vi "GeoFonu_v1.3.vi"() -> ()   [LabVIEW 2014]
uses:
  <vilib>/Instr/_visa.llb/VISA Set IO Buffer Mask.ctl
  <vilib>/Instr/_visa.llb/VISA Flush IO Buffer Mask.ctl
  <vilib>/Instr/_visa.llb/VISA Configure Serial Port (Instr).vi
panel:
  out "Sensor3":i32[](graph)=[342, 333, 338, 337, 336, 340, 338, 334, 337, 337, 333, 337, 339, 337, 337, 337, 317, 337, 334, 335, 338, 338, 316, 333, 339, 337, 338, 337, 338, 337, 337, 338, 335, 334, 338, 334, 337, 337, 338, 337, 337, 339, 335, 338, 337, 338, 337, 336, 334, 332, 338, 335, 337, 335, 334, 337, 337, 335, 338, 338, 335, 336, 338, 337, 337, 336, 337, 339, 337, 336, 338, 337, 337, 335, 334, 335, 337, 338, 329, 338, 337, 338, 339, 339, 335, 338, 337, 334, 351, 337, 328, 346, 336, 337, 336, 339, 336, 338, 335, 333, 337, 360, 338, 333, 338, 334, 339, 336, 336, 337, 336, 313, 339, 337, 337, 337, 304, 338, 338, 338, 336, 340, 336, 336, 338, 335, 338, 335, 338, 333, 329, 336, 342, 336, 335, 335, 338, 336, 336, 338, 334, 336, 336, 313, 337, 337, 334, 329, 338, 336, 329, 341, 336, 335, 336, 338, 332, 334, 337, 336, 336, 337, 334, 337, 336, 333, 336, 336, 338, 336, 337, 338, 342, 338, 344, 338, 343, 338, 338, 325, 336, 337, 337, 335, 338, 339, 337, 339, 336, 336, 336, 336, 332, 334, 338, 338, 339, 359, 339, 333, 337, 339, 333, 338, 337, 338, 336, 342, 338, 336, 336, 337, 334, 337, 337, 341, 335, 334, 338, 335, 341, 333, 336, 336, 330, 335, 336, 336, 331, 340, 336, 337, 334, 336, 336, 334, 341, 334, 336, 339, 338, 336, 336, 336, 335, 335, 336, 336, 337, 334, 336, 335, 339, 336, 334, 334, 338, 336, 338, 334, 338, 336, 334, 337, 336, 339, 336, 338, 334, 334, 336, 336, 335, 335, 336, 335, 333, 336, 336, 338, 337, 333, 336, 337, 351, 335, 337, 336, 337, 336, 334, 336, 341, 334, 360, 336, 339, 339, 336, 336, 338, 333, 338, 329, 334, 326, 338, 339, 339, 339, 336, 337, 335, 341, 335, 339, 340, 337, 336, 337, 341, 331, 336, 336, 326, 336, 339, 339, 337, 335, 337, 335, 334, 335, 337, 338, 336, 335, 335, 336, 337, 336, 343, 337, 335, 329, 336, 359, 336, 334, 338, 345, 336, 336, 333, 337, 337, 336, 339, 338, 331, 337, 335, 336, 338, 332, 343, 338, 341, 329, 337, 339, 333, 331, 336, 342, 338, 337, 337, 336, 336, 338, 331, 334, 336, 337, 336, 338, 336, 335, 336, 336, 336, 331, 336, 335, 334, 338, 337, 338, 338, 336, 334, 333, 337, 335, 343, 328, 339, 338, 349, 336, 334, 336, 336, 342, 339, 334, 338, 337, 336, 334, 336, 340, 340, 339, 346, 338, 337, 338, 337, 340, 336, 328, 338, 335, 338, 338, 337, 338, 338, 336, 337, 334, 338, 344, 339, 336, 339, 338, 338, 336, 336, 340, 295, 338, 337, 334, 336, 337, 337, 336, 336, 336, 338, 340, 339, 336, 341, 339, 361, 337, 336, 336, 338, 339, 335, 337, 336, 340, 338, 336, 338, 336, 338, 339, 339, 336, 334, 333, 337, 338, 336, 338, 334, 339, 336, 337, 335, 335, 336, 338, 339, 337, 334, 336, 336, 334, 352, 337, 336, 336, 338, 339, 334, 338, 336, 335, 336, 336, 336, 335, 336, 337, 336, 338, 338, 338, 336, 336, 336, 336, 338, 337, 336, 336, 335, 336, 337, 344, 335, 337, 336, 336, 337, 334, 338, 338, 332, 336, 341, 345, 336, 336, 337, 336, 336, 335, 337, 336, 338, 338, 337, 338, 338, 335, 339, 338, 337, 336, 337, 336, 337, 327, 337, 334, 337, 335, 337, 339, 336, 336, 336, 336, 334, 336, 335, 336, 338, 339, 338, 335, 338, 333, 336, 335, 328, 335, 339, 335, 335, 333, 337, 338, 336, 337, 335, 337, 338, 335, 337, 334, 330, 336, 335, 334, 338, 340, 335, 338, 334, 333, 338, 342, 338, 337, 336, 337, 337, 342, 337, 336, 348, 335, 342, 338, 337, 335, 336, 338, 335, 337, 334, 338, 335, 338, 336, 337, 338, 336, 336, 340, 336, 311, 333, 374, 334, 340, 340, 335, 336, 335, 337, 337, 335, 335, 349, 336, 338, 334, 336, 338, 335, 335, 335, 339, 326, 340, 338, 337, 338, 335, 333, 338, 337, 338, 336, 340, 336, 334, 338, 335, 335, 338, 335]
  out "Sensor2":i32[](graph)=[314, 311, 314, 312, 312, 311, 308, 313, 311, 313, 311, 312, 315, 311, 309, 311, 311, 317, 271, 313, 309, 314, 311, 312, 313, 313, 315, 313, 312, 301, 311, 314, 309, 311, 313, 311, 313, 313, 311, 314, 315, 313, 314, 316, 311, 312, 311, 314, 311, 311, 311, 317, 312, 312, 310, 312, 311, 311, 312, 314, 309, 313, 314, 312, 311, 311, 311, 314, 311, 311, 309, 311, 311, 310, 314, 315, 311, 311, 309, 314, 312, 289, 311, 312, 309, 312, 312, 313, 315, 309, 311, 310, 315, 312, 312, 310, 309, 314, 313, 310, 313, 313, 313, 310, 308, 305, 312, 303, 314, 313, 314, 313, 311, 312, 311, 311, 311, 314, 305, 313, 308, 311, 311, 304, 312, 304, 309, 314, 310, 312, 310, 312, 314, 311, 313, 336, 310, 312, 312, 310, 313, 306, 314, 314, 312, 313, 313, 313, 309, 316, 313, 317, 311, 316, 310, 311, 313, 307, 314, 310, 314, 313, 310, 315, 312, 311, 311, 313, 312, 311, 313, 310, 311, 310, 314, 291, 311, 312, 310, 309, 313, 313, 311, 320, 314, 312, 312, 316, 308, 296, 312, 313, 312, 313, 313, 311, 311, 313, 312, 313, 300, 311, 313, 313, 292, 313, 312, 313, 313, 311, 311, 313, 318, 310, 311, 312, 310, 310, 313, 314, 313, 316, 313, 313, 314, 309, 316, 310, 314, 312, 311, 311, 313, 312, 313, 311, 308, 310, 313, 311, 313, 308, 312, 310, 318, 311, 310, 313, 313, 318, 309, 313, 311, 311, 311, 313, 314, 312, 313, 306, 313, 310, 311, 310, 310, 314, 307, 310, 314, 305, 313, 313, 315, 297, 314, 310, 310, 310, 310, 313, 311, 302, 314, 313, 313, 308, 315, 313, 311, 313, 310, 313, 314, 308, 311, 313, 313, 314, 312, 311, 313, 313, 310, 312, 311, 313, 313, 313, 313, 311, 311, 313, 313, 312, 315, 311, 311, 313, 338, 311, 314, 309, 314, 310, 311, 314, 313, 311, 313, 313, 313, 313, 313, 314, 315, 306, 313, 310, 314, 314, 310, 314, 312, 309, 311, 311, 310, 310, 316, 313, 316, 316, 313, 313, 312, 310, 311, 317, 315, 311, 308, 313, 311, 309, 304, 313, 316, 313, 313, 313, 311, 309, 318, 310, 310, 313, 315, 313, 314, 313, 312, 311, 310, 311, 310, 313, 311, 319, 308, 312, 313, 312, 314, 313, 313, 312, 312, 312, 314, 310, 313, 313, 315, 315, 312, 313, 314, 313, 313, 285, 313, 310, 311, 310, 312, 313, 313, 313, 310, 313, 312, 311, 315, 313, 313, 312, 312, 311, 313, 311, 310, 312, 315, 310, 320, 315, 312, 293, 307, 299, 310, 313, 312, 313, 311, 313, 312, 313, 315, 314, 313, 313, 313, 318, 311, 312, 311, 315, 312, 313, 312, 312, 311, 309, 311, 312, 303, 314, 311, 311, 312, 310, 310, 311, 313, 311, 313, 313, 310, 318, 322, 313, 306, 313, 311, 310, 313, 311, 312, 311, 312, 311, 310, 311, 314, 313, 311, 313, 311, 313, 315, 310, 309, 313, 308, 309, 312, 311, 311, 315, 311, 315, 315, 313, 312, 312, 310, 313, 315, 313, 312, 315, 313, 312, 314, 311, 311, 310, 312, 314, 312, 315, 313, 311, 314, 311, 313, 311, 315, 311, 310, 312, 312, 310, 311, 313, 313, 313, 313, 312, 312, 312, 311, 313, 311, 311, 311, 311, 311, 312, 313, 313, 311, 307, 312, 311, 311, 313, 313, 313, 311, 313, 312, 311, 313, 311, 312, 309, 313, 311, 311, 312, 314, 312, 312, 329, 311, 314, 308, 313, 314, 312, 310, 312, 309, 312, 311, 314, 310, 308, 312, 312, 330, 311, 309, 314, 313, 313, 310, 312, 315, 313, 312, 311, 312, 315, 310, 313, 312, 309, 311, 312, 309, 308, 312, 306, 313, 312, 311, 314, 312, 312, 311, 315, 311, 312, 313, 314, 312, 312, 310, 311, 291, 315, 313, 312, 309, 311, 312, 313, 311, 315, 301, 310, 314, 312, 311, 314, 312, 315, 312, 312, 311, 311, 311, 306, 307, 319, 311, 314, 312, 312, 312, 312, 315, 310, 311, 313, 305, 310, 313, 311, 313, 310, 314, 314, 314, 311, 292, 311, 311, 312, 312, 315, 312]
  out "Sensor1":i32[](graph)=[315, 315, 312, 311, 315, 315, 317, 317, 318, 314, 318, 321, 316, 315, 318, 318, 317, 318, 319, 318, 317, 315, 315, 317, 316, 315, 317, 315, 316, 317, 326, 319, 329, 314, 315, 317, 316, 316, 314, 318, 311, 316, 317, 317, 317, 314, 317, 316, 318, 319, 315, 317, 317, 316, 314, 317, 316, 315, 317, 316, 317, 319, 319, 316, 312, 304, 282, 317, 316, 317, 314, 317, 318, 317, 319, 316, 317, 315, 316, 319, 315, 317, 316, 317, 314, 320, 294, 325, 315, 316, 301, 318, 318, 317, 317, 316, 318, 318, 315, 315, 321, 318, 316, 315, 320, 316, 321, 312, 319, 319, 315, 315, 316, 309, 316, 317, 314, 315, 315, 314, 317, 318, 317, 316, 316, 318, 315, 316, 316, 318, 320, 322, 315, 315, 313, 315, 315, 287, 315, 313, 316, 315, 303, 315, 317, 315, 320, 317, 318, 317, 318, 317, 316, 318, 320, 316, 313, 314, 324, 326, 318, 318, 316, 316, 307, 317, 318, 316, 315, 314, 318, 315, 318, 313, 317, 315, 316, 316, 316, 316, 316, 314, 317, 323, 318, 318, 315, 316, 313, 316, 318, 305, 317, 323, 317, 318, 316, 315, 316, 318, 318, 314, 319, 316, 316, 282, 317, 315, 318, 316, 319, 317, 317, 315, 298, 319, 315, 320, 317, 316, 318, 314, 315, 314, 315, 316, 317, 316, 315, 318, 316, 318, 316, 315, 318, 316, 318, 315, 315, 315, 315, 318, 313, 317, 304, 317, 311, 316, 316, 315, 315, 315, 315, 317, 290, 317, 318, 315, 317, 316, 315, 318, 314, 316, 320, 319, 316, 317, 314, 317, 317, 316, 315, 316, 314, 306, 317, 315, 320, 316, 314, 314, 320, 318, 317, 318, 318, 318, 317, 317, 326, 316, 316, 316, 315, 318, 317, 338, 318, 316, 315, 318, 313, 316, 311, 318, 316, 320, 315, 315, 316, 283, 317, 316, 314, 318, 316, 308, 316, 318, 314, 316, 316, 315, 316, 315, 318, 316, 320, 319, 317, 316, 311, 315, 315, 313, 321, 313, 318, 317, 316, 316, 316, 317, 319, 317, 317, 313, 315, 314, 314, 317, 314, 315, 318, 316, 316, 316, 318, 316, 316, 318, 318, 303, 317, 317, 315, 317, 315, 318, 318, 317, 317, 317, 315, 316, 318, 319, 316, 316, 316, 315, 313, 306, 315, 312, 318, 316, 318, 318, 314, 313, 313, 315, 313, 318, 314, 317, 317, 348, 318, 284, 315, 315, 312, 315, 317, 316, 314, 316, 316, 314, 313, 303, 316, 318, 319, 317, 316, 317, 319, 313, 315, 308, 316, 317, 318, 308, 314, 316, 317, 318, 316, 318, 327, 313, 314, 315, 313, 315, 316, 318, 318, 312, 307, 316, 315, 313, 318, 316, 319, 326, 313, 317, 315, 305, 316, 316, 314, 319, 318, 316, 316, 312, 315, 314, 315, 314, 318, 316, 315, 318, 315, 317, 315, 319, 317, 314, 315, 317, 316, 339, 316, 317, 321, 318, 317, 315, 315, 316, 316, 317, 316, 315, 316, 320, 317, 317, 316, 316, 317, 315, 310, 316, 317, 316, 316, 315, 316, 317, 316, 316, 316, 316, 348, 314, 315, 317, 318, 314, 318, 317, 316, 316, 316, 318, 317, 316, 316, 318, 318, 314, 316, 316, 315, 315, 317, 316, 318, 318, 313, 318, 316, 318, 316, 313, 313, 314, 318, 316, 315, 318, 314, 318, 315, 316, 315, 317, 316, 316, 316, 317, 316, 310, 317, 316, 315, 318, 318, 315, 316, 315, 316, 316, 313, 316, 318, 317, 323, 316, 315, 316, 317, 316, 317, 316, 314, 316, 317, 328, 315, 316, 325, 315, 315, 312, 312, 317, 335, 317, 315, 316, 319, 316, 317, 314, 315, 320, 317, 315, 317, 312, 314, 313, 319, 316, 313, 319, 315, 318, 314, 316, 315, 314, 315, 315, 317, 317, 312, 314, 317, 317, 317, 315, 319, 317, 317, 315, 343, 309, 316, 316, 316, 315, 317, 318, 314, 314, 314, 318, 316, 314, 317, 316, 315, 312, 315, 318, 317, 311, 316, 320, 314, 317, 316, 317, 318, 314, 315, 317, 312, 315, 326, 317, 299, 316, 317, 316, 316, 317, 314, 312, 303, 316, 315, 315, 315, 313, 319, 314, 314, 312, 317, 319, 318]
  in  "milliseconds to wait":u32=500
  in  "stop":bool
  in  "VISA resource name":refnum<visa-resource-name>
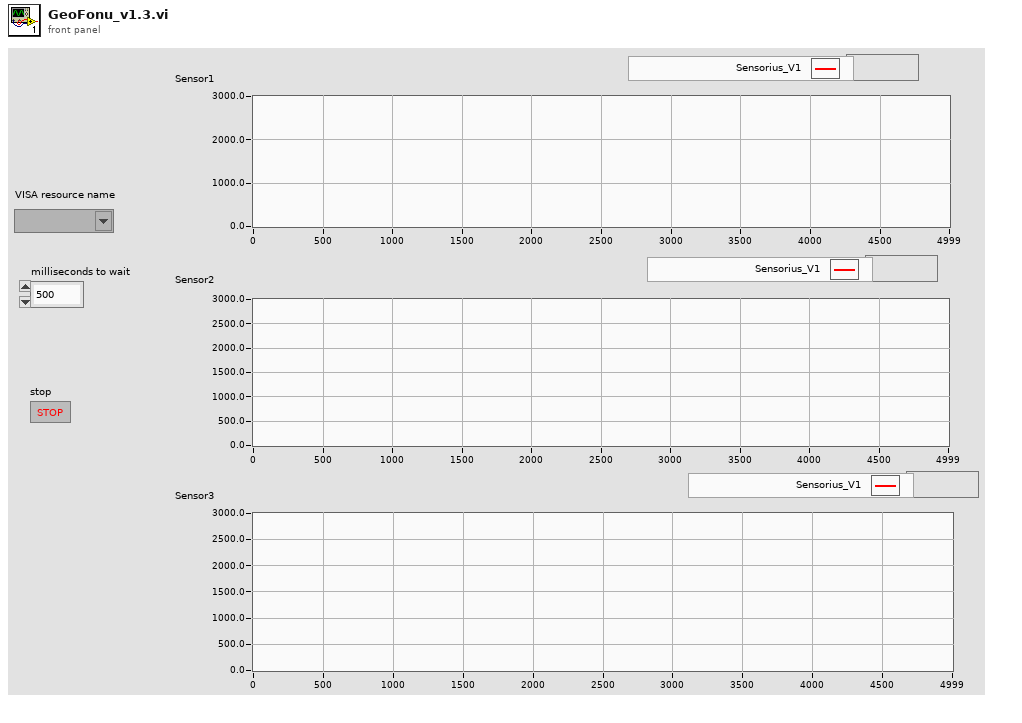
[diagram p1: front panel]
types:
  T1 = typedef "VISA Set IO Buffer Mask.ctl" = u16
  T2 = typedef "VISA Flush IO Buffer Mask.ctl" = u16
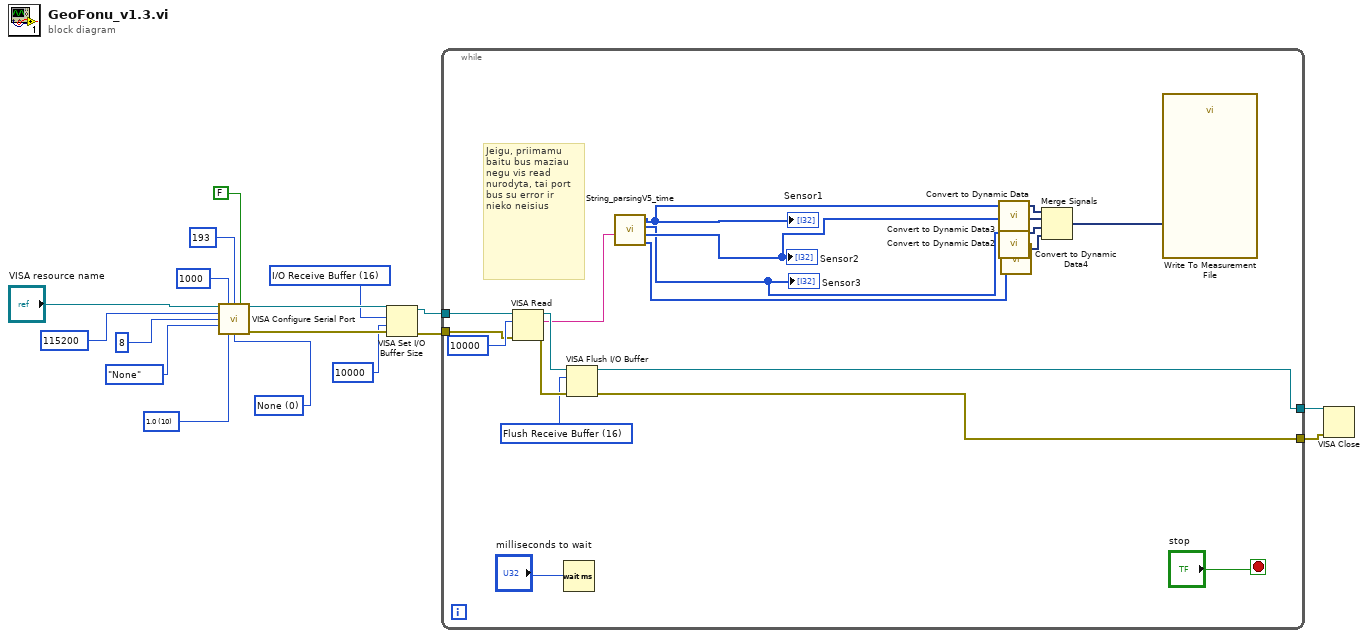
[diagram p0: block diagram]
diagram:
  w7 = T1 16 items=["I/O Receive Buffer"=16, "I/O Transmit Buffer"=32, "I/O Receive and Transmit Buffer"=48] ("Mask")
  w13 = u16 0 items=["None", "XON/XOFF", "RTS/CTS", "XON/XOFF & RTS/CTS", "DTR/DSR", "XON/XOFF & DTR/DSR"] ("flow control (0:none)")
  w14 = u16 10 items=["1.0"=10, "1.5"=15, "2.0"=20] ("stop bits (10: 1 bit)")
  n1 = call-poly "VISA Configure Serial Port"("VISA resource name"="VISA resource name", "timeout (10sec)"=u32 1000, "termination char\n(0xA = '\\n' = LF)"=u8 193 ("termination char\n(0xA = '\\n' = LF)"), "Enable Termination\nChar (T)"=FALSE ("Enable Termination\nChar (T)"), "baud rate (9600)"=u32 115200, "data bits (8)"=u16 8, "parity (0:none)"=enum16{"None", "Odd", "Even", "Mark", "Space"}."None", "stop bits (10: 1 bit)"=w14, "flow control (0:none)"=w13) -> ("VISA resource name out"=w9:refnum<visa-resource-name>, "error out"=w10:errorcluster)  [unwired: 5 in]
  n2 = VISA Set I/O Buffer Size(VISA resource name=w9, mask (16)=w7, size (4096)=u32 10000, error in (no error)=w10) -> (VISA resource name out=w3:refnum<visa-resource-name>, error out=w6:errorcluster)
  n3 = while {
    tunnel: w3 -> [w37]
    tunnel: w6 -> [w34]
    tunnel: [w29] -> w2
    tunnel: [w28] -> w1
    stop <- "stop" stop-if-true
    w31 = T2 16 items=["Flush Receive Buffer"=16, "Write Transmit Buffer to Device"=32, "Flush Receive Buffer (No I/O)"=64, "Flush Transmit Buffer"=128] ("Mask")
    # "Jeigu, priimamu baitu bus maziau negu vis read nurodyta, tai port bus su error ir nieko neisius"
    n4 = VISA Read(VISA resource name=w37, byte count=u32 10000, error in (no error)=w34) -> (VISA resource name out=w33:refnum<visa-resource-name>, read buffer=w23:string, error out=w32:errorcluster)  [unwired: 1 out]
    n5 = Wait (ms)(milliseconds to wait="milliseconds to wait") -> ()  [unwired: 1 out]
    n6 = VISA Flush I/O Buffer(VISA resource name=w33, mask (16)=w31, error in (no error)=w32) -> (VISA resource name out=w29:refnum<visa-resource-name>, error out=w28:errorcluster)
    n7 = call "String_parsingV5_time.vi"("input string"=w23) -> ("Time"=w19:i32[], "V2"=w21:i32[], "V3"=w20:i32[], "V1"=w22:i32[])  [unwired: 3 in]
    "Sensor1" <- w22
    "Sensor2" <- w21
    "Sensor3" <- w20
    n8 = call "Convert to Dynamic Data"("Array"=w22) -> ("Dynamic Data Type"=w27:dynamicdata)  [unwired: 3 in]
    n9 = call "Convert to Dynamic Data3"("Array"=w21) -> ("Dynamic Data Type"=w24:dynamicdata)  [unwired: 3 in]
    n10 = call "Convert to Dynamic Data2"("Array"=w20) -> ("Dynamic Data Type"=w25:dynamicdata)  [unwired: 3 in]
    n11 = call "Convert to Dynamic Data4"("Array"=w19) -> ("Dynamic Data Type"=w18:dynamicdata)  [unwired: 3 in]
    n12 = Merge Signals(w27, w24, w25, w18) -> (w26:dynamicdata)
    n13 = call "Write To Measurement File"("Signals"=w26) -> ()  [unwired: 16 in, 3 out]
  }
  n14 = VISA Close(VISA resource name=w2, error in (no error)=w1) -> ()  [unwired: 1 out]
